vi "Untitled 1.vi"() -> ()   [LabVIEW 2018]
panel:
  out "Boolean":bool
  out "Numeric 2":dbl
  in  "Numeric":dbl
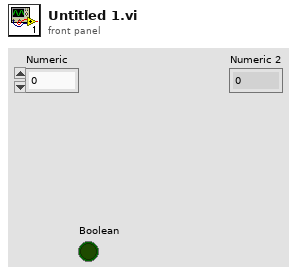
[diagram p1: front panel]
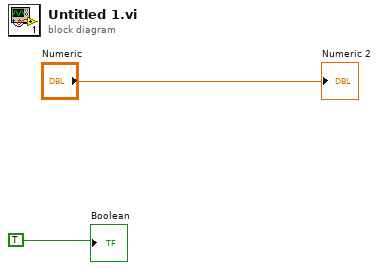
[diagram p0: block diagram]
diagram:
  "Numeric 2" <- "Numeric"
  "Boolean" <- TRUE
